vi "RPM of wheel.vi"() -> ()   [LabVIEW 2016]
panel:
  out "RPM":dbl
  in  "Radius (inches)":dbl
  in  "Second":dbl
  in  "REV":dbl
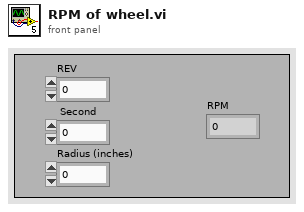
[diagram p1: front panel]
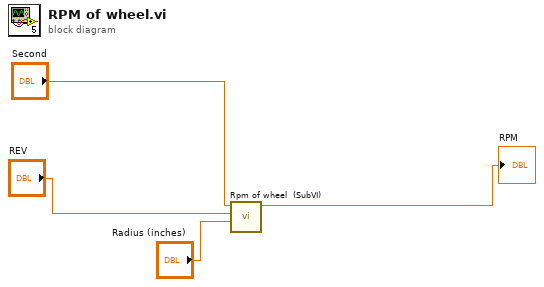
[diagram p0: block diagram]
diagram:
  n1 = call "Rpm of wheel  (SubVI).vi"("Radius (inches)"="Radius (inches)", "REV"="REV", "Second"="Second") -> ("RPM"=→"RPM":dbl)  [unwired: 8 in]
